vi "Stop Core.vi"(10 "final error code":i32, 11 "LS218 in":refnum<class "LS218.lvclass">) -> (3 "LS218 out":refnum<class "LS218.lvclass">)   [LabVIEW 2015, in "LS218.lvlib" / "LS218.lvclass"]
doc: "(<B>Filename</B>: Actor Framework.lvlib:Actor.lvclass:Stop Core.vi)\n\nDefines what the actor does before it stops. Use the <B>final error code</B> input to determine whether the actor shut down in response to an error.\n\nBy default, this method does nothing. A descendant class may override it to define behavior, such as shutting down any processes the actor initiated in its override of the Actor Core method."
uses:
  LS218.lvclass
  LS218.lvclass/LS218.ctl
  CSPP_Core/Actors/CS++DeviceActor/CS++DeviceActor.lvclass
  CSPP_Core/Classes/CS++ProcessVariables/PVConnection/PVConnection.lvclass
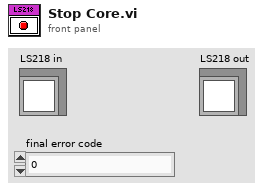
[diagram p1: front panel]
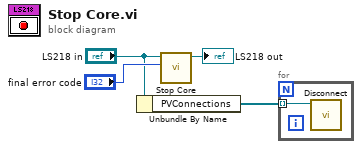
[diagram p0: block diagram]
diagram:
  n1 = Unbundle By Name("LS218 in") -> ("PVConnections"=w1:refnum<class "PVConnection.lvclass">[])
  n2 = call-parent "Stop Core.vi"("final error code"="final error code", "CS++DeviceActor in"="LS218 in") -> ("CS++DeviceActor out"=→"LS218 out":refnum<class "LS218.lvclass">)  [unwired: 9 in]
  n3 = for {
    tunnel: w1 -> [w5] mode=indexing
    n4 = call "Disconnect.vi"("PVConnection in"=w5) -> ()  [unwired: 9 in, 2 out]
  }
